vi "optionsAcq_attenuator.vi"(6 "poll write":bool, 8 "error in (no error)":errorcluster, 9 "readWrite":enum16{"read", "write"}(ring), 10 "attenuator":bool, 11 "Thorlabs_OSA200_64 in":refnum<class "OSA200.lvclass">) -> (0 "error out":errorcluster, 1 "status":string, 2 "attenuator out":bool, 3 "Thorlabs_OSA200_64 out":refnum<class "OSA200.lvclass">, 4 "poll timeOut":bool)   [LabVIEW 2010, in "OSA200.lvclass"]
uses:
  OSA200.lvclass
  OSA.lvclass
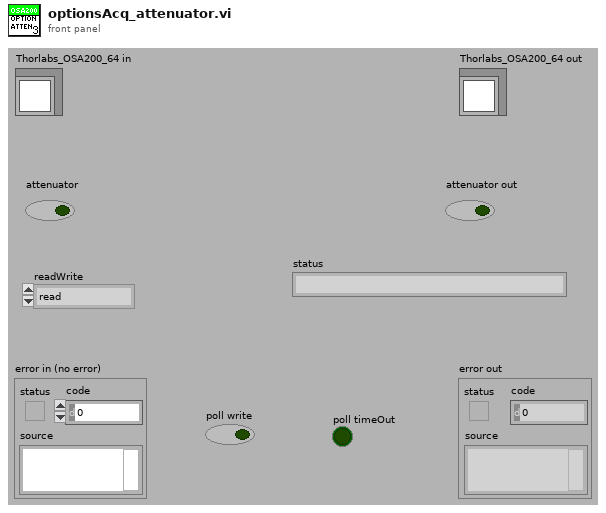
[diagram p1: front panel]
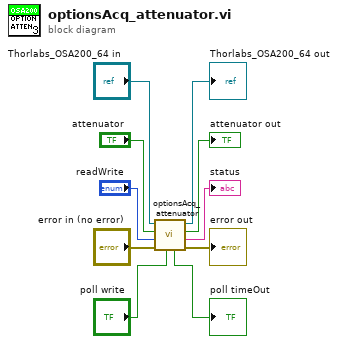
[diagram p0: block diagram]
diagram:
  n1 = call-parent "optionsAcq_attenuator.vi"("poll write"="poll write", "error in (no error)"="error in (no error)", "readWrite"="readWrite", "attenuator"="attenuator", "Thorlabs_OSA_64 in"="Thorlabs_OSA200_64 in") -> ("error out"=→"error out":errorcluster, "status"=→"status":string, "attenuator out"=→"attenuator out":bool, "Thorlabs_OSA_64 out"=→"Thorlabs_OSA200_64 out":refnum<class "OSA200.lvclass">, "poll timeOut"=→"poll timeOut":bool)  [unwired: 2 in]
